vi "test Get-Set-Get Default Word Value.vi"(8 "error in":errorcluster, 11 "TestCase in":refnum<class "Scripting.lvclass">) -> (0 "error out":errorcluster, 3 "TestCase out":refnum<class "Scripting.lvclass">)   [LabVIEW 2020, in "Scripting.lvclass"]
uses:
  Scripting.lvclass
  Scripting.lvclass/Scripting.ctl
  <vilib>/addons/_JKI Toolkits/VI Tester/TestCase.llb/TestCase.lvclass
  Scripting/Communication Bus Template Scripting.lvlib
  C:/Program Files (x86)/National Instruments/LabVIEW 2020/vi.lib/addons/_JKI Toolkits/VI Tester/TestCase.llb/TestCase.lvclass
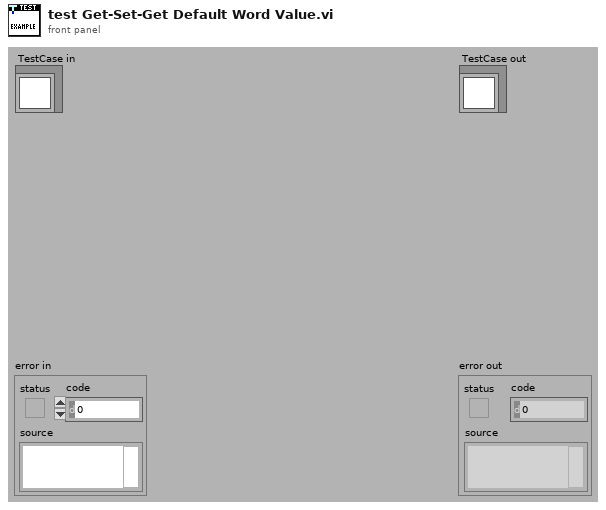
[diagram p1: front panel]
types:
  T1 = typedef "Custom Device API.lvlib/Custom Device Item Ref.ctl" = u64
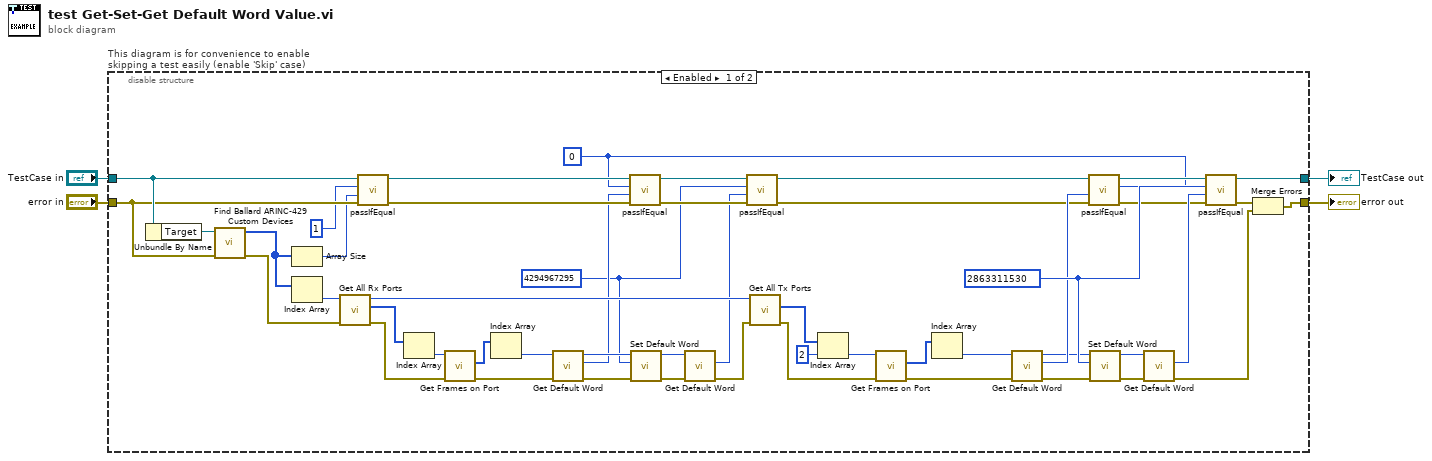
[diagram p0: block diagram]
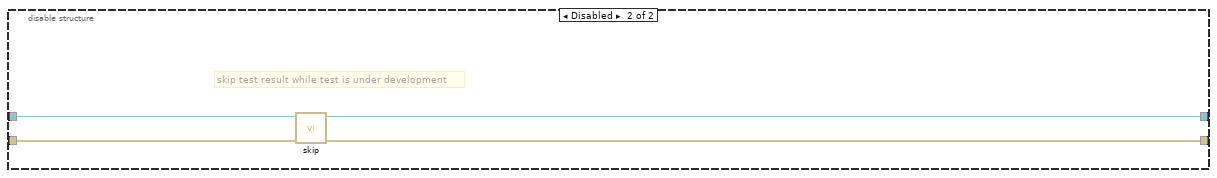
[diagram p2: hidden frame]
diagram:
  n1 = disable-structure "This diagram is for convenience to enable skipping a test easily (enable 'Skip' case)" shown="Enabled" {
    disable-tunnel: "TestCase in" -> [w52 w58]
    disable-tunnel: [w6 w56] -> w1
    disable-tunnel: [w42 w57] -> w3
    disable-tunnel: "error in" -> [w51 w55]
    frame Enabled {
      w20 = u32 2863311530 ("default word")
      w24 = u32 4294967295 ("default word")
      w5 = u32 0 ("default word")
      n2 = Unbundle By Name(w52) -> ("Target"=w54:refnum<k24>)
      n3 = call "Find Ballard ARINC-429 Custom Devices.vi"("error in"=w51, "target"=w54) -> ("error out"=w46:errorcluster, "Ballard ARINC-429 custom devices"=w50:u64[])  [unwired: 8 in]
      n4 = Array Size(array=w50) -> (size(s)=w48:i32)
      n5 = Index Array(array=w50) -> (element=w53:u64)  [unwired: 1 in]
      n6 = call "Get All Rx Ports.vi"("error in"=w46, "Ballard ARINC 429 custom device in"=w53) -> ("error out"=w40:errorcluster, "Rx hardware channel refs"=w47:T1[], "Ballard ARINC 429 custom device out"=w45:T1)  [unwired: 7 in]
      n7 = call-dynamic "passIfEqual.vi"("error in (no error)"=w51, "y"=w48, "x"=1 ("size(s)"), "TestCase in"=w52) -> ("error out"=w28:errorcluster, "TestCase out"=w29:refnum<class "Scripting.lvclass">)  [unwired: 6 in]
      n8 = Index Array(array=w47) -> (element=w41:T1)  [unwired: 1 in]
      n9 = call "Get Frames on Port.vi"("error in"=w40, "port ref in"=w41) -> ("error out"=w35:errorcluster, "frame references"=w36:T1[])  [unwired: 6 in, 2 out]
      n10 = Index Array(array=w36) -> (element=w34:T1)  [unwired: 1 in]
      n11 = call "Get Default Word.vi"("error in"=w35, "Item Ref in"=w34) -> ("error out"=w33:errorcluster, "default word"=w27:u32, "Item Ref out"=w32:T1)  [unwired: 7 in]
      n12 = call-dynamic "passIfEqual.vi"("error in (no error)"=w28, "y"=w27, "x"=w5, "TestCase in"=w29) -> ("error out"=w25:errorcluster, "TestCase out"=w26:refnum<class "Scripting.lvclass">)  [unwired: 6 in]
      n13 = call "Set Default Word.vi"("error in"=w33, "default word"=w24, "Item Ref in"=w32) -> ("error out"=w31:errorcluster, "Item Ref out"=w30:T1)  [unwired: 7 in]
      n14 = call "Get Default Word.vi"("error in"=w31, "Item Ref in"=w30) -> ("error out"=w22:errorcluster, "default word"=w23:u32)  [unwired: 7 in, 1 out]
      n15 = call-dynamic "passIfEqual.vi"("error in (no error)"=w25, "y"=w23, "x"=w24, "TestCase in"=w26) -> ("error out"=w13:errorcluster, "TestCase out"=w9:refnum<class "Scripting.lvclass">)  [unwired: 6 in]
      n16 = call "Get All Tx Ports.vi"("error in"=w22, "Ballard ARINC 429 custom device in"=w45) -> ("error out"=w39:errorcluster, "Tx hardware channel refs"=w44:T1[])  [unwired: 7 in, 1 out]
      n17 = Index Array(array=w44, index=2) -> (element=w38:T1)
      n18 = call "Get Frames on Port.vi"("error in"=w39, "port ref in"=w38) -> ("error out"=w12:errorcluster, "frame references"=w37:T1[])  [unwired: 6 in, 2 out]
      n19 = Index Array(array=w37) -> (element=w11:T1)  [unwired: 1 in]
      n20 = call "Get Default Word.vi"("error in"=w12, "Item Ref in"=w11) -> ("error out"=w14:errorcluster, "default word"=w18:u32, "Item Ref out"=w15:T1)  [unwired: 7 in]
      n21 = call-dynamic "passIfEqual.vi"("error in (no error)"=w13, "y"=w18, "x"=w5, "TestCase in"=w9) -> ("error out"=w19:errorcluster, "TestCase out"=w8:refnum<class "Scripting.lvclass">)  [unwired: 6 in]
      n22 = call "Set Default Word.vi"("error in"=w14, "default word"=w20, "Item Ref in"=w15) -> ("error out"=w16:errorcluster, "Item Ref out"=w17:T1)  [unwired: 7 in]
      n23 = call "Get Default Word.vi"("error in"=w16, "Item Ref in"=w17) -> ("error out"=w10:errorcluster, "default word"=w21:u32)  [unwired: 7 in, 1 out]
      n24 = call-dynamic "passIfEqual.vi"("error in (no error)"=w19, "y"=w21, "x"=w20, "TestCase in"=w8) -> ("error out"=w7:errorcluster, "TestCase out"=w6:refnum<class "Scripting.lvclass">)  [unwired: 6 in]
      n25 = Merge Errors(w7, w10) -> (w42:errorcluster)
    }
    frame Disabled {
      # "skip test result while test is under development"
      n26 = call <vilib>:"skip.vi"("error in (no error)"=w55, "TestCase in"=w58) -> ("error out"=w57:errorcluster, "TestCase out"=w56:refnum<class "Scripting.lvclass">)  [unwired: 8 in]
    }
  }
  "error out" <- w3
  "TestCase out" <- w1
